vi "VisionNetwork.vi"(8 "error in (no error)":errorcluster) -> (0 "error out":errorcluster)   [LabVIEW 2023]
doc: "Vision Network\n\nInput\n --Error in \n\nOutput\n --Error out"
uses:
  VisionGlobal.vi
  <vilib>/Rock Robotics/Network Tables/NT Write Number.vi
  <vilib>/Rock Robotics/Network Tables/NT Write Boolean.vi
  <vilib>/Rock Robotics/Network Tables/NT Write Integer.vi
  <vilib>/Rock Robotics/WPI/ThirdParty/JAS_Junk/TrajLib/Trajectory_Library.lvlib
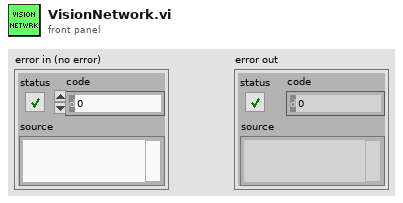
[diagram p1: front panel]
types:
  T1 = typedef "Trajectory_Library.lvlib/POSE2D.ctl" = cluster{"TRANSLATION":T2, "ROTATION":T3}
  T2 = typedef "Trajectory_Library.lvlib/TRANSLATION2D.ctl" = cluster{"X":dbl, "Y":dbl}
  T3 = typedef "Trajectory_Library.lvlib/ROTATION2D.ctl" = cluster{"VALUE":dbl, "COS":dbl, "SIN":dbl}
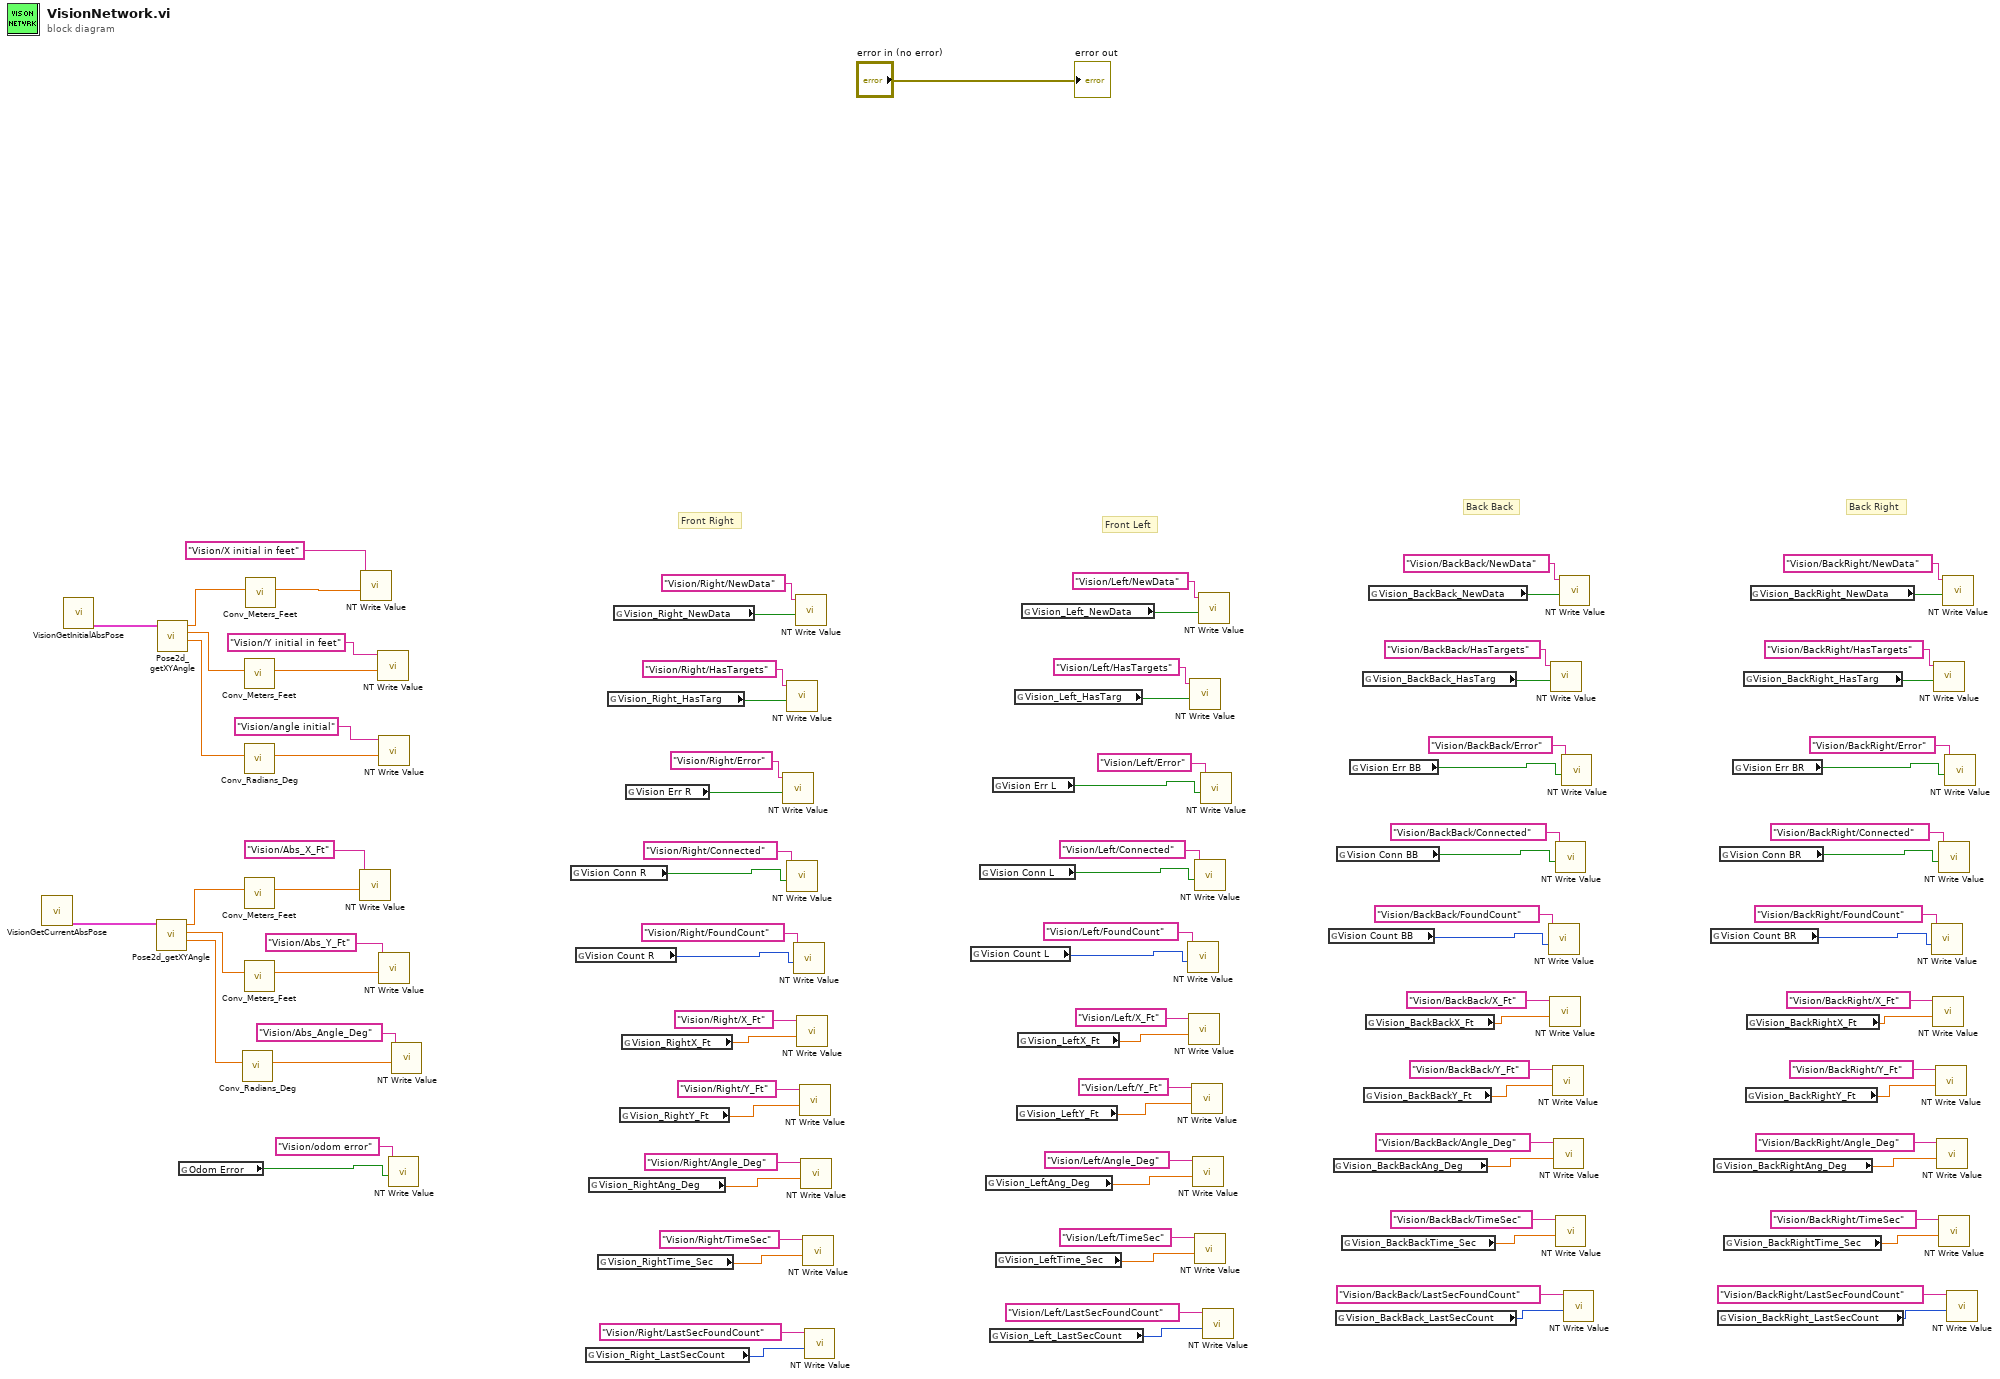
[diagram p0: block diagram]
diagram:
  # "Back Right"
  # "Back Back"
  # "Front Left"
  # "Front Right"
  n1 = call "VisionGetCurrentAbsPose.vi"() -> ("Current ABS Pose"=w102:T1)  [unwired: 9 in]
  n2 = call "VisionGetInitialAbsPose.vi"() -> ("InitialABSPose"=w89:T1)  [unwired: 10 in]
  n3 = call <vilib>:"Pose2d_getXYAngle.vi"("in POSE"=w102) -> ("Angle"=w101:dbl, "Y"=w100:dbl, "X"=w99:dbl)  [unwired: 8 in]
  n4 = call <vilib>:"Pose2d_getXYAngle.vi"("in POSE"=w89) -> ("Angle"=w95:dbl, "Y"=w94:dbl, "X"=w93:dbl)  [unwired: 8 in]
  n5 = global read "VisionGlobal.vi" "Odom Error"() -> (w81:bool)
  n6 = call <vilib>:"Conv_Radians_Deg.vi"("Radians"=w101) -> ("Degrees"=w96:dbl)  [unwired: 10 in]
  n7 = call <vilib>:"Conv_Meters_Feet.vi"("Meters"=w94) -> ("Feet"=w91:dbl)  [unwired: 10 in]
  n8 = call <vilib>:"Conv_Radians_Deg.vi"("Radians"=w95) -> ("Degrees"=w90:dbl)  [unwired: 10 in]
  n9 = call <vilib>:"Conv_Meters_Feet.vi"("Meters"=w99) -> ("Feet"=w98:dbl)  [unwired: 10 in]
  n10 = call <vilib>:"Conv_Meters_Feet.vi"("Meters"=w100) -> ("Feet"=w97:dbl)  [unwired: 10 in]
  n11 = call <vilib>:"Conv_Meters_Feet.vi"("Meters"=w93) -> ("Feet"=w92:dbl)  [unwired: 10 in]
  n12 = call-poly <vilib>:"NT Write Value.vi"("value"=w98, "name"="Vision/Abs_X_Ft") -> ()  [unwired: 9 in, 1 out]
  n13 = call-poly <vilib>:"NT Write Value.vi"("value"=w92, "name"="Vision/X initial in feet") -> ()  [unwired: 9 in, 1 out]
  n14 = call-poly <vilib>:"NT Write Value.vi"("value"=w91, "name"="Vision/Y initial in feet") -> ()  [unwired: 9 in, 1 out]
  n15 = call-poly <vilib>:"NT Write Value.vi"("value"=w90, "name"="Vision/angle initial") -> ()  [unwired: 9 in, 1 out]
  n16 = call-poly <vilib>:"NT Write Value.vi"("value"=w97, "name"="Vision/Abs_Y_Ft") -> ()  [unwired: 9 in, 1 out]
  n17 = call-poly <vilib>:"NT Write Value.vi"("value"=w81, "name"="Vision/odom error") -> ()  [unwired: 9 in, 1 out]
  n18 = call-poly <vilib>:"NT Write Value.vi"("value"=w96, "name"="Vision/Abs_Angle_Deg") -> ()  [unwired: 9 in, 1 out]
  n19 = global read "VisionGlobal.vi" "Vision Conn R"() -> (w72:bool)
  n20 = global read "VisionGlobal.vi" "Vision Count R"() -> (w70:i32)
  n21 = global read "VisionGlobal.vi" "Vision_Right_LastSecCount"() -> (w43:i32)
  n22 = global read "VisionGlobal.vi" "Vision_RightAng_Deg"() -> (w61:dbl)
  n23 = global read "VisionGlobal.vi" "Vision_RightTime_Sec"() -> (w64:dbl)
  n24 = global read "VisionGlobal.vi" "Vision_Right_HasTarg"() -> (w52:bool)
  n25 = global read "VisionGlobal.vi" "Vision_Right_NewData"() -> (w50:bool)
  n26 = global read "VisionGlobal.vi" "Vision_RightY_Ft"() -> (w62:dbl)
  n27 = global read "VisionGlobal.vi" "Vision_RightX_Ft"() -> (w63:dbl)
  n28 = global read "VisionGlobal.vi" "Vision Err R"() -> (w74:bool)
  n29 = call-poly <vilib>:"NT Write Value.vi"("value"=w74, "name"="Vision/Right/Error") -> ()  [unwired: 9 in, 1 out]
  n30 = call-poly <vilib>:"NT Write Value.vi"("value"=w52, "name"="Vision/Right/HasTargets") -> ()  [unwired: 9 in, 1 out]
  n31 = call-poly <vilib>:"NT Write Value.vi"("value"=w72, "name"="Vision/Right/Connected") -> ()  [unwired: 9 in, 1 out]
  n32 = call-poly <vilib>:"NT Write Value.vi"("value"=w70, "name"="Vision/Right/FoundCount") -> ()  [unwired: 9 in, 1 out]
  n33 = call-poly <vilib>:"NT Write Value.vi"("value"=w50, "name"="Vision/Right/NewData") -> ()  [unwired: 9 in, 1 out]
  n34 = call-poly <vilib>:"NT Write Value.vi"("value"=w63, "name"="Vision/Right/X_Ft") -> ()  [unwired: 9 in, 1 out]
  n35 = call-poly <vilib>:"NT Write Value.vi"("value"=w62, "name"="Vision/Right/Y_Ft") -> ()  [unwired: 9 in, 1 out]
  n36 = call-poly <vilib>:"NT Write Value.vi"("value"=w61, "name"="Vision/Right/Angle_Deg") -> ()  [unwired: 9 in, 1 out]
  n37 = call-poly <vilib>:"NT Write Value.vi"("value"=w64, "name"="Vision/Right/TimeSec") -> ()  [unwired: 9 in, 1 out]
  n38 = call-poly <vilib>:"NT Write Value.vi"("value"=w43, "name"="Vision/Right/LastSecFoundCount") -> ()  [unwired: 9 in, 1 out]
  n39 = global read "VisionGlobal.vi" "Vision Count L"() -> (w79:i32)
  n40 = global read "VisionGlobal.vi" "Vision Conn L"() -> (w75:bool)
  n41 = global read "VisionGlobal.vi" "Vision_LeftAng_Deg"() -> (w53:dbl)
  n42 = global read "VisionGlobal.vi" "Vision_Left_LastSecCount"() -> (w41:i32)
  n43 = global read "VisionGlobal.vi" "Vision Err L"() -> (w77:bool)
  n44 = global read "VisionGlobal.vi" "Vision_LeftTime_Sec"() -> (w56:dbl)
  n45 = global read "VisionGlobal.vi" "Vision_Left_HasTarg"() -> (w48:bool)
  n46 = global read "VisionGlobal.vi" "Vision_LeftY_Ft"() -> (w54:dbl)
  n47 = global read "VisionGlobal.vi" "Vision_LeftX_Ft"() -> (w55:dbl)
  n48 = global read "VisionGlobal.vi" "Vision_Left_NewData"() -> (w46:bool)
  n49 = call-poly <vilib>:"NT Write Value.vi"("value"=w79, "name"="Vision/Left/FoundCount") -> ()  [unwired: 9 in, 1 out]
  n50 = call-poly <vilib>:"NT Write Value.vi"("value"=w55, "name"="Vision/Left/X_Ft") -> ()  [unwired: 9 in, 1 out]
  n51 = call-poly <vilib>:"NT Write Value.vi"("value"=w48, "name"="Vision/Left/HasTargets") -> ()  [unwired: 9 in, 1 out]
  n52 = call-poly <vilib>:"NT Write Value.vi"("value"=w54, "name"="Vision/Left/Y_Ft") -> ()  [unwired: 9 in, 1 out]
  n53 = call-poly <vilib>:"NT Write Value.vi"("value"=w53, "name"="Vision/Left/Angle_Deg") -> ()  [unwired: 9 in, 1 out]
  n54 = call-poly <vilib>:"NT Write Value.vi"("value"=w75, "name"="Vision/Left/Connected") -> ()  [unwired: 9 in, 1 out]
  n55 = call-poly <vilib>:"NT Write Value.vi"("value"=w56, "name"="Vision/Left/TimeSec") -> ()  [unwired: 9 in, 1 out]
  n56 = call-poly <vilib>:"NT Write Value.vi"("value"=w46, "name"="Vision/Left/NewData") -> ()  [unwired: 9 in, 1 out]
  n57 = call-poly <vilib>:"NT Write Value.vi"("value"=w77, "name"="Vision/Left/Error") -> ()  [unwired: 9 in, 1 out]
  n58 = call-poly <vilib>:"NT Write Value.vi"("value"=w41, "name"="Vision/Left/LastSecFoundCount") -> ()  [unwired: 9 in, 1 out]
  n59 = global read "VisionGlobal.vi" "Vision Count BB"() -> (w39:i32)
  n60 = global read "VisionGlobal.vi" "Vision_BackBackAng_Deg"() -> (w27:dbl)
  n61 = global read "VisionGlobal.vi" "Vision_BackBack_LastSecCount"() -> (w21:i32)
  n62 = global read "VisionGlobal.vi" "Vision Conn BB"() -> (w35:bool)
  n63 = global read "VisionGlobal.vi" "Vision_BackBackTime_Sec"() -> (w30:dbl)
  n64 = global read "VisionGlobal.vi" "Vision Err BB"() -> (w37:bool)
  n65 = global read "VisionGlobal.vi" "Vision_BackBack_HasTarg"() -> (w26:bool)
  n66 = global read "VisionGlobal.vi" "Vision_BackBackY_Ft"() -> (w28:dbl)
  n67 = global read "VisionGlobal.vi" "Vision_BackBackX_Ft"() -> (w29:dbl)
  n68 = global read "VisionGlobal.vi" "Vision_BackBack_NewData"() -> (w24:bool)
  n69 = call-poly <vilib>:"NT Write Value.vi"("value"=w39, "name"="Vision/BackBack/FoundCount") -> ()  [unwired: 9 in, 1 out]
  n70 = call-poly <vilib>:"NT Write Value.vi"("value"=w29, "name"="Vision/BackBack/X_Ft") -> ()  [unwired: 9 in, 1 out]
  n71 = call-poly <vilib>:"NT Write Value.vi"("value"=w26, "name"="Vision/BackBack/HasTargets") -> ()  [unwired: 9 in, 1 out]
  n72 = call-poly <vilib>:"NT Write Value.vi"("value"=w28, "name"="Vision/BackBack/Y_Ft") -> ()  [unwired: 9 in, 1 out]
  n73 = call-poly <vilib>:"NT Write Value.vi"("value"=w27, "name"="Vision/BackBack/Angle_Deg") -> ()  [unwired: 9 in, 1 out]
  n74 = call-poly <vilib>:"NT Write Value.vi"("value"=w35, "name"="Vision/BackBack/Connected") -> ()  [unwired: 9 in, 1 out]
  n75 = call-poly <vilib>:"NT Write Value.vi"("value"=w30, "name"="Vision/BackBack/TimeSec") -> ()  [unwired: 9 in, 1 out]
  n76 = call-poly <vilib>:"NT Write Value.vi"("value"=w24, "name"="Vision/BackBack/NewData") -> ()  [unwired: 9 in, 1 out]
  n77 = call-poly <vilib>:"NT Write Value.vi"("value"=w37, "name"="Vision/BackBack/Error") -> ()  [unwired: 9 in, 1 out]
  n78 = call-poly <vilib>:"NT Write Value.vi"("value"=w21, "name"="Vision/BackBack/LastSecFoundCount") -> ()  [unwired: 9 in, 1 out]
  n79 = global read "VisionGlobal.vi" "Vision Count BR"() -> (w19:i32)
  n80 = global read "VisionGlobal.vi" "Vision_BackRightAng_Deg"() -> (w7:dbl)
  n81 = global read "VisionGlobal.vi" "Vision_BackRight_LastSecCount"() -> (w1:i32)
  n82 = global read "VisionGlobal.vi" "Vision Conn BR"() -> (w15:bool)
  n83 = global read "VisionGlobal.vi" "Vision_BackRightTime_Sec"() -> (w10:dbl)
  n84 = global read "VisionGlobal.vi" "Vision Err BR"() -> (w17:bool)
  n85 = global read "VisionGlobal.vi" "Vision_BackRight_HasTarg"() -> (w6:bool)
  n86 = global read "VisionGlobal.vi" "Vision_BackRightY_Ft"() -> (w8:dbl)
  n87 = global read "VisionGlobal.vi" "Vision_BackRightX_Ft"() -> (w9:dbl)
  n88 = global read "VisionGlobal.vi" "Vision_BackRight_NewData"() -> (w4:bool)
  n89 = call-poly <vilib>:"NT Write Value.vi"("value"=w19, "name"="Vision/BackRight/FoundCount") -> ()  [unwired: 9 in, 1 out]
  n90 = call-poly <vilib>:"NT Write Value.vi"("value"=w9, "name"="Vision/BackRight/X_Ft") -> ()  [unwired: 9 in, 1 out]
  n91 = call-poly <vilib>:"NT Write Value.vi"("value"=w6, "name"="Vision/BackRight/HasTargets") -> ()  [unwired: 9 in, 1 out]
  n92 = call-poly <vilib>:"NT Write Value.vi"("value"=w8, "name"="Vision/BackRight/Y_Ft") -> ()  [unwired: 9 in, 1 out]
  n93 = call-poly <vilib>:"NT Write Value.vi"("value"=w7, "name"="Vision/BackRight/Angle_Deg") -> ()  [unwired: 9 in, 1 out]
  n94 = call-poly <vilib>:"NT Write Value.vi"("value"=w15, "name"="Vision/BackRight/Connected") -> ()  [unwired: 9 in, 1 out]
  n95 = call-poly <vilib>:"NT Write Value.vi"("value"=w10, "name"="Vision/BackRight/TimeSec") -> ()  [unwired: 9 in, 1 out]
  n96 = call-poly <vilib>:"NT Write Value.vi"("value"=w4, "name"="Vision/BackRight/NewData") -> ()  [unwired: 9 in, 1 out]
  n97 = call-poly <vilib>:"NT Write Value.vi"("value"=w17, "name"="Vision/BackRight/Error") -> ()  [unwired: 9 in, 1 out]
  n98 = call-poly <vilib>:"NT Write Value.vi"("value"=w1, "name"="Vision/BackRight/LastSecFoundCount") -> ()  [unwired: 9 in, 1 out]
  "error out" <- "error in (no error)"
